vi "multinumericlimittest1.vi"(4 "Sequence Context":T1) -> (0 "error out":errorcluster, 1 "Test Data":T2 {"Numeric Measurement" format="%.2f"})   [LabVIEW 2011]
uses:
  Demo/LabVIEW/SupportVIs.llb/LabVIEW Test - Test Data.ctl
  <vilib>/addons/TestStand/_TSLegacy.llb/LabVIEW Test - Sequence Context.ctl
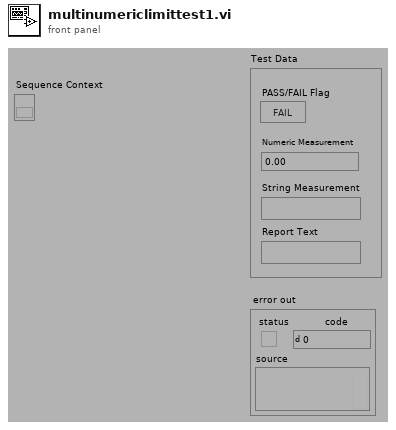
[diagram p1: front panel]
types:
  T1 = typedef "LabVIEW Test - Sequence Context.ctl" = refnum<k7>
  T2 = typedef "LabVIEW Test - Test Data.ctl" = cluster{"PASS/FAIL Flag":bool, "Numeric Measurement":dbl, "String Measurement":string, "Report Text":string}
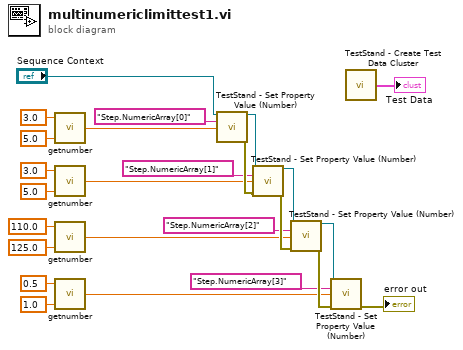
[diagram p0: block diagram]
diagram:
  n1 = call "getnumber.vi"("High Limit"=5.0, "Low Limit"=3.0) -> ("Numeric"=w4:dbl)  [unwired: 3 out]
  n2 = call "getnumber.vi"("High Limit"=5.0, "Low Limit"=3.0) -> ("Numeric"=w5:dbl)  [unwired: 3 out]
  n3 = call "getnumber.vi"("High Limit"=125.0, "Low Limit"=110.0) -> ("Numeric"=w8:dbl)  [unwired: 3 out]
  n4 = call "getnumber.vi"("High Limit"=1.0, "Low Limit"=0.5) -> ("Numeric"=w10:dbl)  [unwired: 3 out]
  n5 = call <vilib>:"TestStand - Set Property Value (Number).vi"("Sequence Context In"="Sequence Context", "Lookup String"="Step.NumericArray[0]", "New Value"=w4) -> ("Sequence Context Out"=w16:refnum<k7>, "error out"=w13:errorcluster)  [unwired: 2 in, 9 out]
  n6 = call <vilib>:"TestStand - Set Property Value (Number).vi"("Sequence Context In"=w16, "Lookup String"="Step.NumericArray[1]", "New Value"=w5, "error in (no error)"=w13) -> ("Sequence Context Out"=w15:refnum<k7>, "error out"=w12:errorcluster)  [unwired: 1 in, 9 out]
  n7 = call <vilib>:"TestStand - Set Property Value (Number).vi"("Sequence Context In"=w15, "Lookup String"="Step.NumericArray[2]", "New Value"=w8, "error in (no error)"=w12) -> ("Sequence Context Out"=w14:refnum<k7>, "error out"=w11:errorcluster)  [unwired: 1 in, 9 out]
  n8 = call <vilib>:"TestStand - Set Property Value (Number).vi"("Sequence Context In"=w14, "Lookup String"="Step.NumericArray[3]", "New Value"=w10, "error in (no error)"=w11) -> ("error out"=→"error out":errorcluster)  [unwired: 1 in, 10 out]
  n9 = call "TestStand - Create Test Data Cluster.vi"() -> ("Test Data"=→"Test Data":T2)  [unwired: 4 in]
